vi "Select DLP Device & Get COM.vi"(8 "error in (no error)":errorcluster, 11 "Device Type Selection":enum16{"IOR4 device", "IO20 device"}(ring)) -> (0 "error out":errorcluster, 2 "Selected device":T1, 3 "Selected COM":refnum<visa-resource-name>)   [LabVIEW 2020, in "DLP Design Modules Driver.lvlib"]
uses:
  DLP Design Modules Driver.lvlib
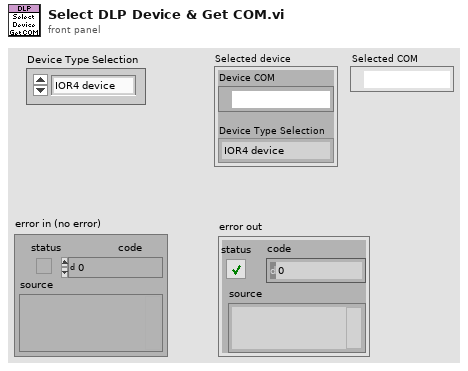
[diagram p1: front panel]
types:
  T1 = cluster{"Device COM":refnum<visa-resource-name>, "Device Type Selection":enum16{"IOR4 device", "IO20 device"}}
  T2 = cluster{"Device COM":refnum<visa-resource-name>, "Device Type":enum16{"IOR4 device", "IO20 device"}}[]
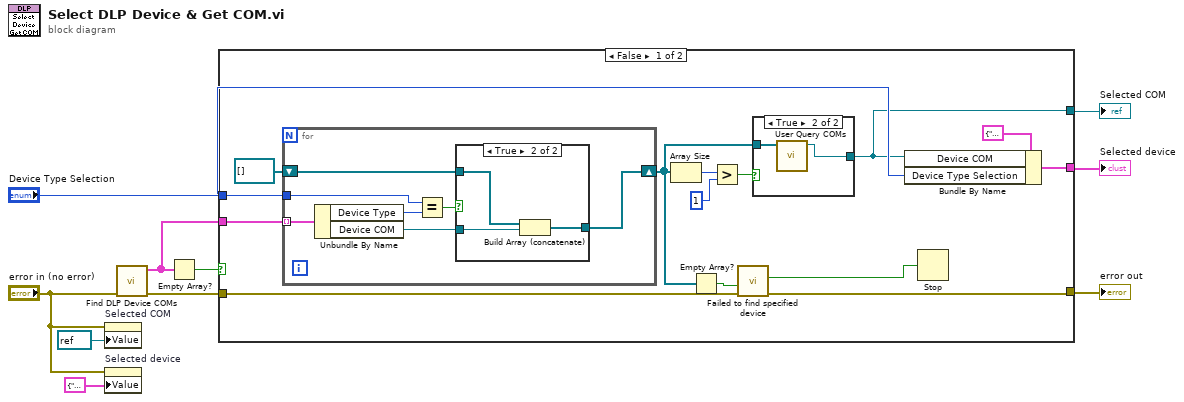
[diagram p0: block diagram]
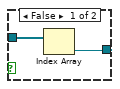
[diagram p2: hidden frame]
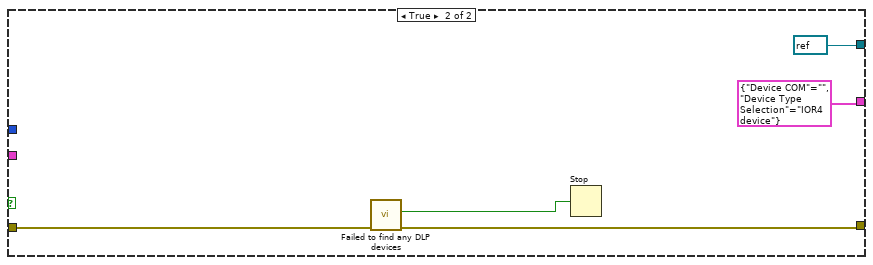
[diagram p4: hidden frame]
diagram:
  n1 = property on="Selected COM" class="VISAName"(error in="error in (no error)", "Value"=refnum<visa-resource-name> refnum ("Device COM")) -> ()  [unwired: 1 in, 2 out]
  n2 = property on="Selected device" class="Clust (strict)"(error in="error in (no error)", "Value"=T1 {"Device COM"="", "Device Type Selection"=enum."IOR4 device"} ("input cluster")) -> ()  [unwired: 1 in, 2 out]
  n3 = call "Find DLP Device COMs.vi"("error in (no error)"="error in (no error)") -> ("error out"=w9:errorcluster, "DLP COMs"=w8:T2)  [unwired: 7 in]
  n4 = Empty Array?(array=w8) -> (empty?=w10:bool)
  n5 = case shown="False" w10 {
    tunnel: w9 -> [w13 w44]
    tunnel: w8 -> [w24 _]
    tunnel: "Device Type Selection" -> [w20 _]
    tunnel: [w18 refnum<visa-resource-name> refnum ("Device COM")] -> w4
    tunnel: [w12 w43] -> w6
    tunnel: [w17 T1 {"Device COM"="", "Device Type Selection"=enum."IOR4 device"} ("input cluster")] -> w5
    frame False {
      n6 = for {
        tunnel: w24 -> [w35] mode=indexing
        tunnel: w20 -> [w33]
        shift-right: [w29] -> w15
        shift-left: refnum<visa-resource-name>[] [] -> [w30]
        n7 = Unbundle By Name(w35) -> ("Device Type"=w34:enum16{"IOR4 device", "IO20 device"}, "Device COM"=w31:refnum<visa-resource-name>)
        n8 = Equal?(x=w33, y=w34) -> (x = y?=w32:bool)
        n9 = case shown="True" w32 {
          tunnel: w31 -> [_ w39]
          tunnel: w30 -> [w36 w38]
          tunnel: [w36 w37] -> w29
          frame False {
          }
          frame True {
            n10 = Build Array (concatenate)(w38, w39) -> (w37:refnum<visa-resource-name>[])
          }
        }
      }
      n11 = Array Size(array=w15) -> (size(s)=w23:i32)
      n12 = Empty Array?(array=w15) -> (empty?=w14:bool)
      n13 = Greater?(x=w23, y=1) -> (0:w21:bool)
      n14 = call "Failed to find specified device"("error in (no error)"=w13, "Enable"=w14) -> ("error out"=w12:errorcluster, "OK"=w11:bool)  [unwired: 8 in]
      n15 = case shown="True" w21 {
        tunnel: w15 -> [w26 w28]
        tunnel: [w25 w27] -> w18
        frame False {
          n16 = Index Array(array=w26) -> (element=w25:refnum<visa-resource-name>)  [unwired: 1 in]
        }
        frame True {
          n17 = call "User Query COMs.vi"("COMs"=w28) -> ("Selected COM"=w27:refnum<visa-resource-name>)  [unwired: 10 in]
        }
      }
      n18 = Bundle By Name(cluster=T1 {"Device COM"="", "Device Type Selection"=enum."IOR4 device"} ("input cluster"), "Device COM"=w18, "Device Type Selection"=w20) -> (w17:T1)
      n19 = Stop(stop? (T)=w11) -> ()
    }
    frame True {
      n20 = call "Failed to find any DLP devices"("error in (no error)"=w44) -> ("error out"=w43:errorcluster, "OK"=w40:bool)  [unwired: 9 in]
      n21 = Stop(stop? (T)=w40) -> ()
    }
  }
  "error out" <- w6
  "Selected device" <- w5
  "Selected COM" <- w4
